vi "Combine Errors.vi"(1 "error in (no error)":errorcluster, 2 "error in (no error)":errorcluster) -> (0 "error out":errorcluster)   [LabVIEW 2024]
doc: "This VI combines two errors and returns the one that has an actural error status.\nScott Hannahs, <sth@magnet.fsu.edu> NHMFL-FSU, May 2003"
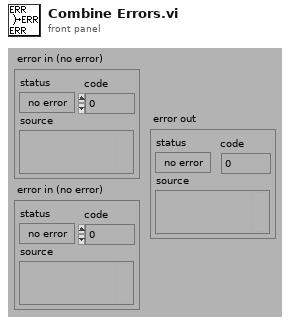
[diagram p1: front panel]
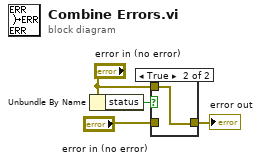
[diagram p0: block diagram]
diagram:
  n1 = Unbundle By Name("error in (no error)") -> ("status"=w2:bool)
  n2 = case shown="True" w2 {
    tunnel: "error in (no error)" -> [w5 _]
    tunnel: [w5 w6] -> w3
    tunnel: "error in (no error)" -> [_ w6]
    frame False {
    }
    frame True {
    }
  }
  "error out" <- w3
